vi "SerialTst.vi"() -> ()   [LabVIEW 2018]
uses:
  Program Files/National Instruments/LabVIEW 2018/examples/Instrument IO/Serial/support/Serial - Settings.ctl
  <vilib>/Instr/_visa.llb/VISA Configure Serial Port (Instr).vi
  SerialGlobal.vi
panel:
  in  "Command":string="+"
  out "Boolean":bool
  out "Response":string
  out "Array":bool[](array[boolean])
  in  "Termination Character":u8=10 format="%.0x"
  in  "End Write on Termination Character?":bool=TRUE
  in  "VISA resource name":refnum<visa-resource-name>="COM4"
  in  "Serial Settings":T1={"baud rate"=9600, "data bits"=8, "parity"=enum."None", "stop bits"=10, "flow control"=0} {"flow control" items=["None"=0, "XON/XOFF"=1, "RTS/CTS"=2, "DTR/DSR"=4]; "stop bits" items=["1.0"=10, "1.5"=15, "2.0"=20]; "data bits" min=5 max=8 step=1; "baud rate" items=["75"=75, "110"=110, "134"=134, "150"=150, "300"=300, "600"=600, "1200"=1200, "1800"=1800, "2400"=2400, "4800"=4800, "7200"=7200, "9600"=9600, "14400"=14400, "19200"=19200, "28800"=28800, "38400"=38400, "56000"=56000, "57600"=57600, "115200"=115200, "128000"=128000, "230400"=230400]}
  in  "End Read on Termination Character?":bool=TRUE
  in  "Stop":bool
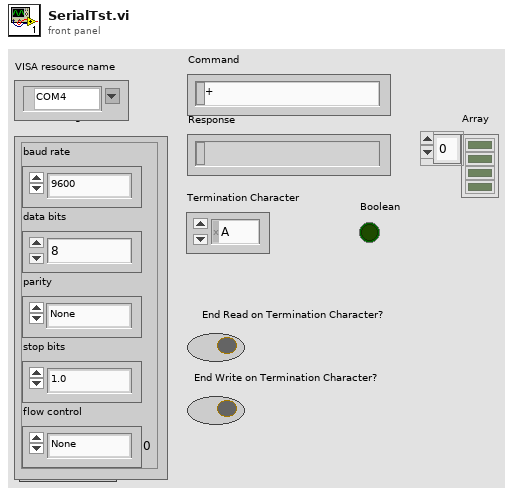
[diagram p1: front panel]
types:
  T1 = typedef "Serial - Settings.ctl" = cluster{"baud rate":u32, "data bits":u16, "parity":enum16{"None", "Odd", "Even", "Mark", "Space"}, "stop bits":u16, "flow control":u16}
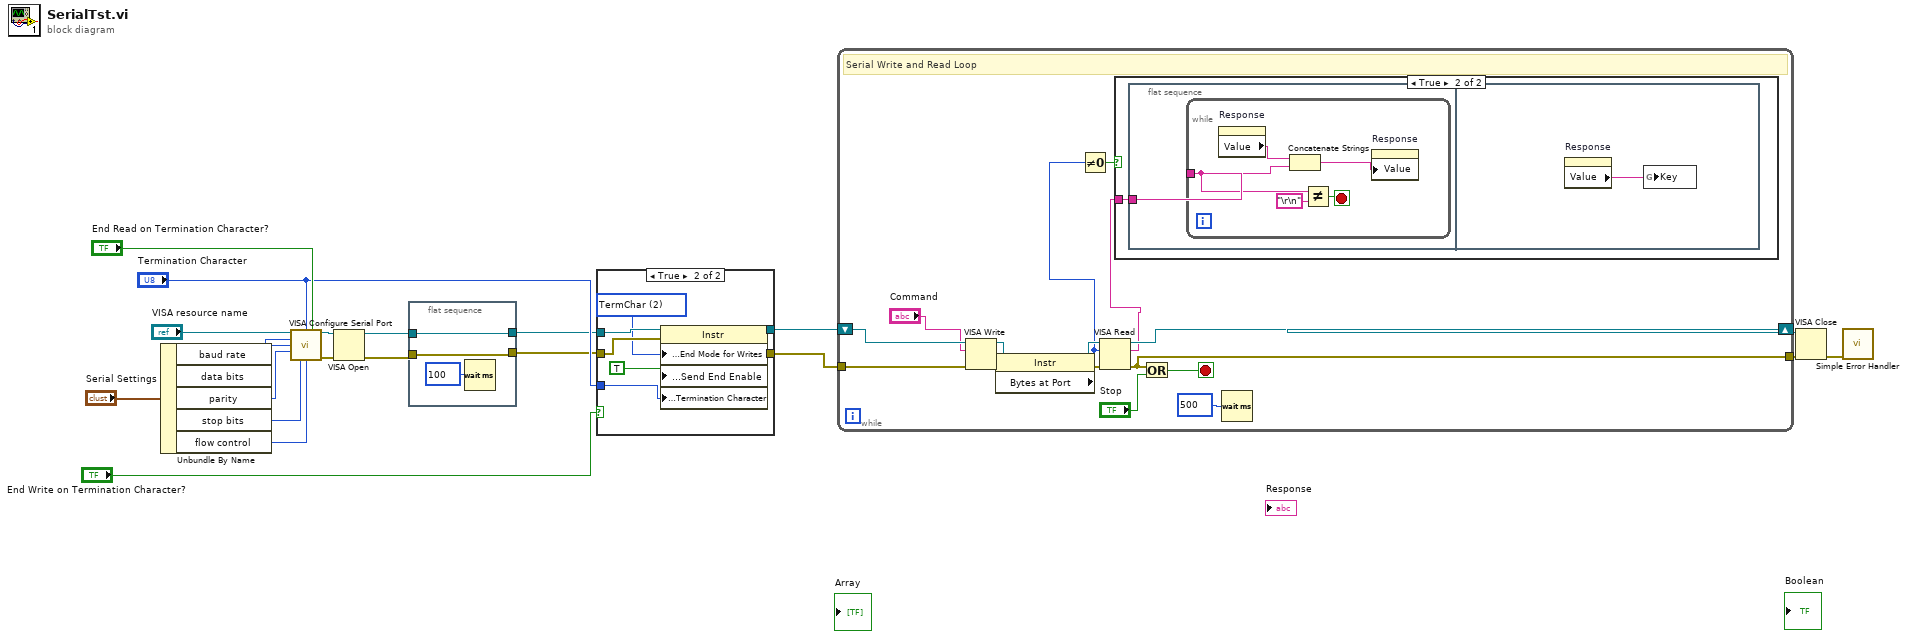
[diagram p0: block diagram]
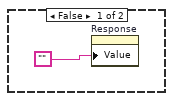
[diagram p3: hidden frame]
diagram:
  n1 = Unbundle By Name("Serial Settings") -> ("baud rate"=w17:u32, "data bits"=w18:u16, "parity"=w19:enum16{"None", "Odd", "Even", "Mark", "Space"}, "stop bits"=w20:u16, "flow control"=w11:u16)
  n2 = call-poly "VISA Configure Serial Port"("VISA resource name"="VISA resource name", "termination char\n(0xA = '\\n' = LF)"="Termination Character", "Enable Termination\nChar (T)"="End Read on Termination Character?", "baud rate (9600)"=w17, "data bits (8)"=w18, "parity (0:none)"=w19, "stop bits (10: 1 bit)"=w20, "flow control (0:none)"=w11) -> ("VISA resource name out"=w6:refnum<visa-resource-name>, "error out"=w5:errorcluster)  [unwired: 2 in, 4 out]
  n3 = VISA Open(error in (no error)=w5, VISA resource name=w6) -> (VISA resource name=w4:refnum<visa-resource-name>, error out=w2:errorcluster)  [unwired: 3 in]
  n4 = flat-sequence {
    tunnel: w4 -> [w24]
    tunnel: [w24] -> w3
    tunnel: [w23] -> w1
    tunnel: w2 -> [w23]
    frame #0 {
      n5 = Wait (ms)(milliseconds to wait=u32 100) -> ()  [unwired: 1 out]
    }
  }
  n6 = case shown="True" "End Write on Termination Character?" {
    tunnel: w3 -> [w25 w33]
    tunnel: w1 -> [w26 w32]
    tunnel: [w25 w31] -> w9
    tunnel: [w26 w30] -> w10
    tunnel: "Termination Character" -> [_ w28]
    frame False {
    }
    frame True {
      w29 = u16 2 items=["None", "LastBit", "TermChar", "Break"] ("Serial Settings:Serial End Mode for Writes")
      n7 = property class="Instr"(reference=w33, error in=w32, "Serial Settings:End Mode for Writes"=w29, "Message Based Settings:Send End Enable"=TRUE, "Message Based Settings:Termination Character"=w28) -> (reference out=w31:refnum<visa-resource-name>, error out=w30:errorcluster)
    }
  }
  n8 = while {
    shift-right: [w48] -> w12
    shift-left: w9 -> [w47]
    tunnel: w10 -> [w46]
    tunnel: [w43] -> w13
    stop <- w44 stop-if-true
    # "Serial Write and Read Loop"
    n9 = VISA Write(VISA resource name=w47, write buffer="Command", error in (no error)=w46) -> (VISA resource name out=w41:refnum<visa-resource-name>, error out=w39:errorcluster)  [unwired: 1 out]
    n10 = property class="Instr"(reference=w41, error in=w39) -> (reference out=w40:refnum<visa-resource-name>, error out=w38:errorcluster, "Bytes at Port"=w37:u32)
    n11 = Not Equal To 0?(x=w37) -> (x != 0?=w35:bool)
    n12 = VISA Read(VISA resource name=w40, byte count=w37, error in (no error)=w38) -> (VISA resource name out=w48:refnum<visa-resource-name>, read buffer=w36:string, error out=w43:errorcluster)  [unwired: 1 out]
    n13 = case shown="True" w35 {
      tunnel: w36 -> [_ w50]
      frame False {
        n14 = property on="Response" class="Str"("Value"="") -> ()  [unwired: 2 in, 2 out]
      }
      frame True {
        n15 = flat-sequence {
          tunnel: w50 -> [w51]
          frame #0 {
            n16 = while {
              tunnel: w51 -> [w55]
              stop <- w56 stop-if-true
              n17 = property on="Response" class="Str"() -> ("Value"=w54:string)  [unwired: 2 in, 2 out]
              n18 = Concatenate Strings(w54, w55) -> (w53:string)
              n19 = Not Equal?(x=w55, y="\r\n") -> (x != y?=w56:bool)
              n20 = property on="Response" class="Str"("Value"=w53) -> ()  [unwired: 2 in, 2 out]
            }
          }
          frame #1 {
            n21 = property on="Response" class="Str"() -> ("Value"=w57:string)  [unwired: 2 in, 2 out]
            n22 = global write "SerialGlobal.vi" "Key"(w57) -> ()
          }
        }
      }
    }
    n23 = Or(x=w43, y="Stop") -> (x .or. y?=w44:bool)
    n24 = Wait (ms)(milliseconds to wait=u32 500) -> ()  [unwired: 1 out]
  }
  n25 = VISA Close(VISA resource name=w12, error in (no error)=w13) -> (error out=w14:errorcluster)
  n26 = call <vilib>:"Simple Error Handler.vi"("error in (no error)"=w14) -> ()  [unwired: 1 in, 8 out]
